vi "Add Entry.vi"(5 "BG Color (None)":u32(colorbox), 6 "Parent (None)":string[](array[string]), 7 "Name Prefix (none)":string, 8 "error in":errorcluster, 9 "Columns":string[](array[string]), 10 "Name":string, 11 "Tree Map in":refnum<class "Tree Map.lvclass">) -> (0 "error out":errorcluster, 3 "Tree Map out":refnum<class "Tree Map.lvclass">, 4 "Hierarchy":string[](array[string]))   [LabVIEW 2020, in "VI Properties Editor.lvlib" / "Tree Map.lvlib" / "Tree Map.lvclass"]
uses:
  Tree Map.lvclass
  Tree Map.lvclass/Tree Map.ctl
  Tree Entry.ctl
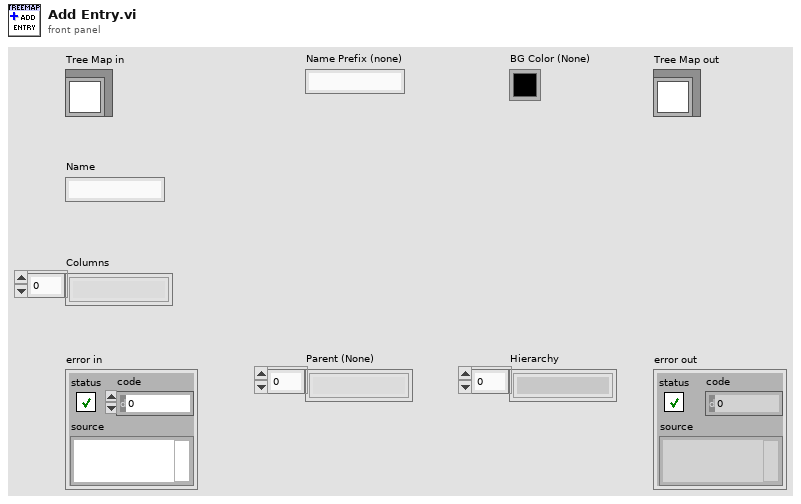
[diagram p1: front panel]
types:
  T1 = typedef "VI Properties Editor.lvlib/Tree Map.lvlib/Tree Map.lvclass/Tree Entry.ctl" = cluster{"Hierarchy":string[], "Name":string, "Columns":string[], "BG Color":u32, "Leaf":bool, "Symbol":string}
  T2 = typedef "imagedata.ctl" = cluster{"image type":i32, "image depth":i32, "image":u8[], "mask":u8[], "colors":u32[], "Rectangle":cluster{"left":i16, "top":i16, "right":i16, "bottom":i16}}
  T3 = map{string, cluster{"index":i32, "image data":T2}}
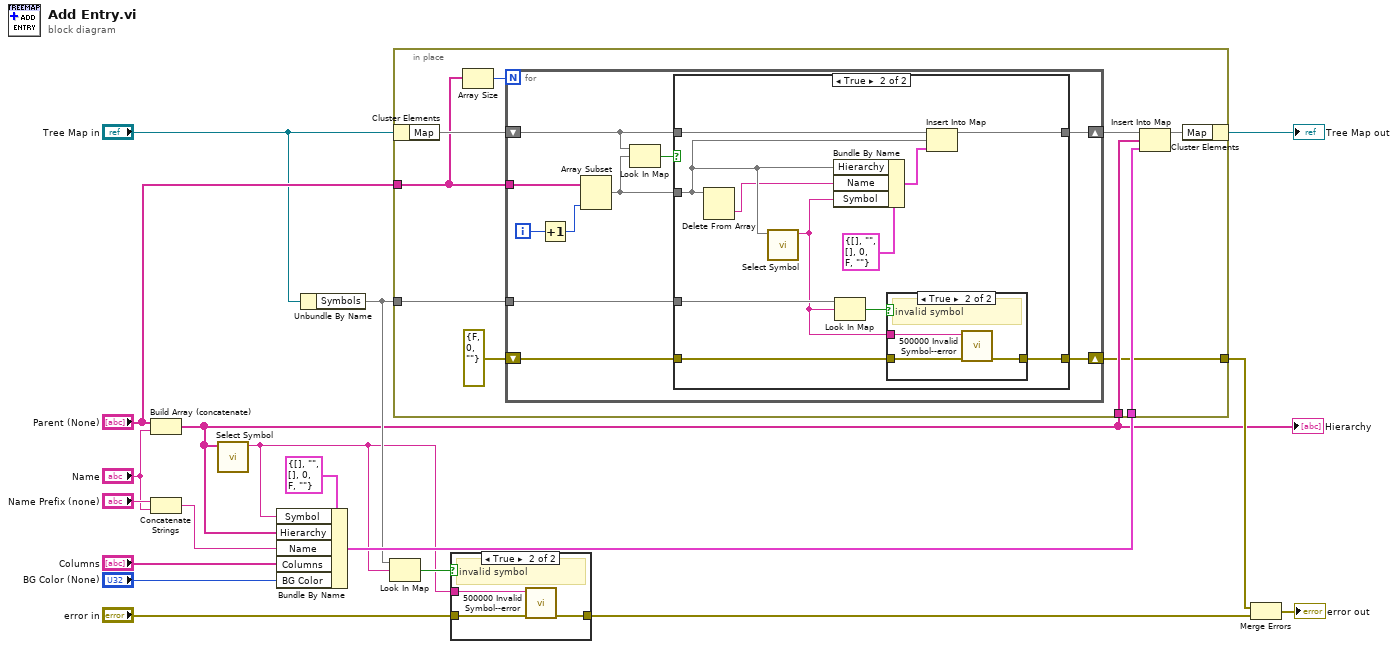
[diagram p0: block diagram]
diagram:
  n1 = Build Array (concatenate)("Parent (None)", "Name") -> (w4:string[])
  "Hierarchy" <- w4
  n2 = Concatenate Strings("Name Prefix (none)", "Name") -> (w16:string)
  n3 = call "Select Symbol.vi"("Hierarchy"=w4) -> ("Symbol ID"=w1:string)  [unwired: 10 in]
  n4 = Bundle By Name(cluster=T1 {"Hierarchy"=[], "Name"="", "Columns"=[], "BG Color"=0, "Leaf"=FALSE, "Symbol"=""} ("Tree Entry"), "Symbol"=w1, "Hierarchy"=w4, "Name"=w16, "Columns"="Columns", "BG Color"="BG Color (None)") -> (w10:T1)
  n5 = Unbundle By Name("Tree Map in") -> ("Symbols"=w5:T3)
  n6 = Look In Map(map=w5, key=w1) -> (key not found?=w2:bool)  [unwired: 1 in, 1 out]
  n7 = in-place {
    in-place-border: w10 -> [w28]
    in-place-border: w4 -> [w27]
    in-place-border: "Parent (None)" -> [w23]
    in-place-border: [w21] -> w6
    in-place-border: w5 -> [w20]
    n8 = in-place-cluster #1("Tree Map in") -> ("Map"=w25:map{string[], T1})
    n9 = Array Size(array=w23) -> (size(s)=w22:i32)
    n10 = for {
      N: w22 -> [_]
      shift-right: [w33] -> w24
      shift-left: w25 -> [w35]
      tunnel: w23 -> [w38]
      tunnel: w20 -> [w30]
      shift-right: [w31] -> w21
      shift-left: errorcluster {"status"=FALSE, "code"=0, "source"=""} ("error out") -> [w29]
      i -> [w37]
      n11 = Increment(x=w37) -> (x+1=w32:i32)
      n12 = Array Subset(array=w38, length=w32) -> (w34:string[])  [unwired: 1 in]
      n13 = Look In Map(map=w35, key=w34) -> (key not found?=w36:bool)  [unwired: 1 in, 1 out]
      n14 = case shown="True" w36 {
        tunnel: w35 -> [w40 w51]
        tunnel: w34 -> [_ w43]
        tunnel: [w40 w50] -> w33
        tunnel: [w39 w45] -> w31
        tunnel: w30 -> [_ w47]
        tunnel: w29 -> [w39 w44]
        frame False {
        }
        frame True {
          n15 = Delete From Array(array=w43) -> (deleted portion=w41:string)  [unwired: 2 in, 1 out]
          n16 = call "Select Symbol.vi"("Hierarchy"=w43) -> ("Symbol ID"=w42:string)  [unwired: 10 in]
          n17 = Bundle By Name(cluster=T1 {"Hierarchy"=[], "Name"="", "Columns"=[], "BG Color"=0, "Leaf"=FALSE, "Symbol"=""} ("value"), "Hierarchy"=w43, "Name"=w41, "Symbol"=w42) -> (w48:T1)
          n18 = Look In Map(map=w47, key=w42) -> (key not found?=w46:bool)  [unwired: 1 in, 1 out]
          n19 = case shown="True" w46 {
            tunnel: [w52 w55] -> w45
            tunnel: w42 -> [_ w54]
            tunnel: w44 -> [w52 w53]
            frame False {
              # "symbol valid"
            }
            frame True {
              # "invalid symbol"
              n20 = call "500000 Invalid Symbol--error.vi"("error in"=w53, "Argument"=w54) -> ("error out"=w55:errorcluster)  [unwired: 8 in, 1 out]
            }
          }
          n21 = Insert Into Map(map in=w51, key=w43, value=w48) -> (map out=w50:map{string[], T1})  [unwired: 2 out]
        }
      }
    }
    n22 = Insert Into Map(map in=w24, key=w27, value=w28) -> (map out=w26:map{string[], T1})  [unwired: 2 out]
    n23 = in-place-cluster #1("Map"=w26) -> (→"Tree Map out":refnum<class "Tree Map.lvclass">)
  }
  n24 = case shown="True" w2 {
    tunnel: "error in" -> [w56 w59]
    tunnel: [w56 w58] -> w9
    tunnel: w1 -> [_ w57]
    frame False {
      # "symbol valid"
    }
    frame True {
      # "invalid symbol"
      n25 = call "500000 Invalid Symbol--error.vi"("error in"=w59, "Argument"=w57) -> ("error out"=w58:errorcluster)  [unwired: 8 in, 1 out]
    }
  }
  n26 = Merge Errors(w6, w9) -> (→"error out":errorcluster)
